vi "Parse Pattern Name.vi"(8 "error in (no error)":errorcluster, 10 "Index":i32, 11 "Pattern Name":string) -> (0 "error out":errorcluster, 3 "Pattern Name out":string)   [LabVIEW 2018, in "Config_Read_BML.lvclass"]
uses:
  Config_Read_BML.lvclass
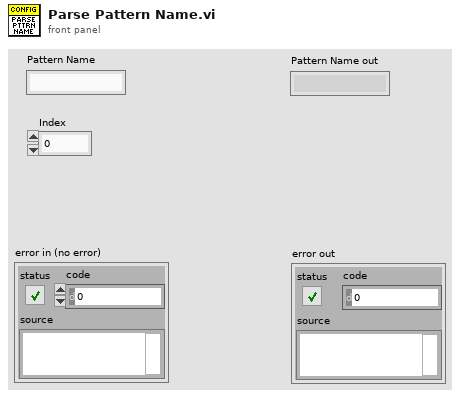
[diagram p1: front panel]
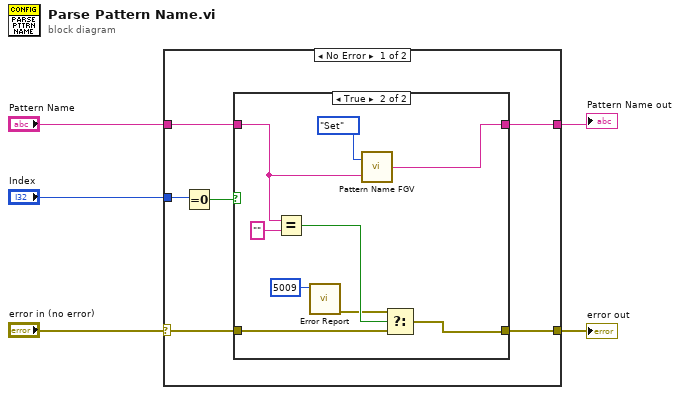
[diagram p0: block diagram]
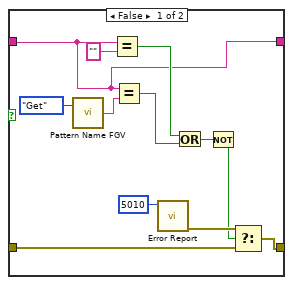
[diagram p2: hidden frame]
diagram:
  n1 = case shown="No Error" "error in (no error)" {
    selector: "error in (no error)" -> [w7 w33]
    tunnel: "Pattern Name" -> [w9 w34]
    tunnel: "Index" -> [w11 _]
    tunnel: [w6 w33] -> w2
    tunnel: [w8 w34] -> w1
    frame No Error {
      n2 = Equal To 0?(x=w11) -> (x = 0?=w10:bool)
      n3 = case shown="True" w10 {
        tunnel: w9 -> [w12 w26]
        tunnel: [w12 w25] -> w8
        tunnel: w7 -> [w16 w29]
        tunnel: [w15 w28] -> w6
        frame False {
          n4 = call "Pattern Name FGV.vi"("Op"=enum16{"Set", "Get"}."Get") -> ("Pattern Name out"=w21:string)  [unwired: 1 in]
          n5 = Equal?(x=w12, y="") -> (x = y?=w20:bool)
          n6 = Equal?(x=w12, y=w21) -> (x = y?=w19:bool)
          n7 = call "Error Report.vi"("Error Code"=i16 5010) -> ("error out"=w18:errorcluster)  [unwired: 10 in]
          n8 = Or(x=w20, y=w19) -> (x .or. y?=w14:bool)
          n9 = Not(x=w14) -> (.not. x?=w13:bool)
          n10 = Select(t=w18, s=w13, f=w16) -> (s? t:f=w15:errorcluster)
        }
        frame True {
          n11 = Equal?(x=w26, y="") -> (x = y?=w31:bool)
          n12 = call "Error Report.vi"("Error Code"=i16 5009) -> ("error out"=w30:errorcluster)  [unwired: 10 in]
          n13 = call "Pattern Name FGV.vi"("String"=w26, "Op"=enum16{"Set", "Get"}."Set") -> ("Pattern Name out"=w25:string)
          n14 = Select(t=w30, s=w31, f=w29) -> (s? t:f=w28:errorcluster)
        }
      }
    }
    frame Error {
    }
  }
  "Pattern Name out" <- w1
  "error out" <- w2
